vi "Simple Moving Average.vi"(9 "Power v time":cluster{dbl[], dbl[]}(graph), 10 "N point average":i32=5) -> (1 "SMA with Time":cluster{dbl[], dbl[]}(graph), 2 "SMA Graph":dbl[](graph))   [LabVIEW 2017]
uses:
  <vilib>/Analysis/baseanly.llb/Mean (DBL).vi
  <vilib>/Analysis/NI_AALBase.lvlib
panel:
  out "Time":dbl[](array[numeric])
  out "Signal In":dbl[](graph)
  # "Data Input"
  # "Local Data"
  # "Data Output"
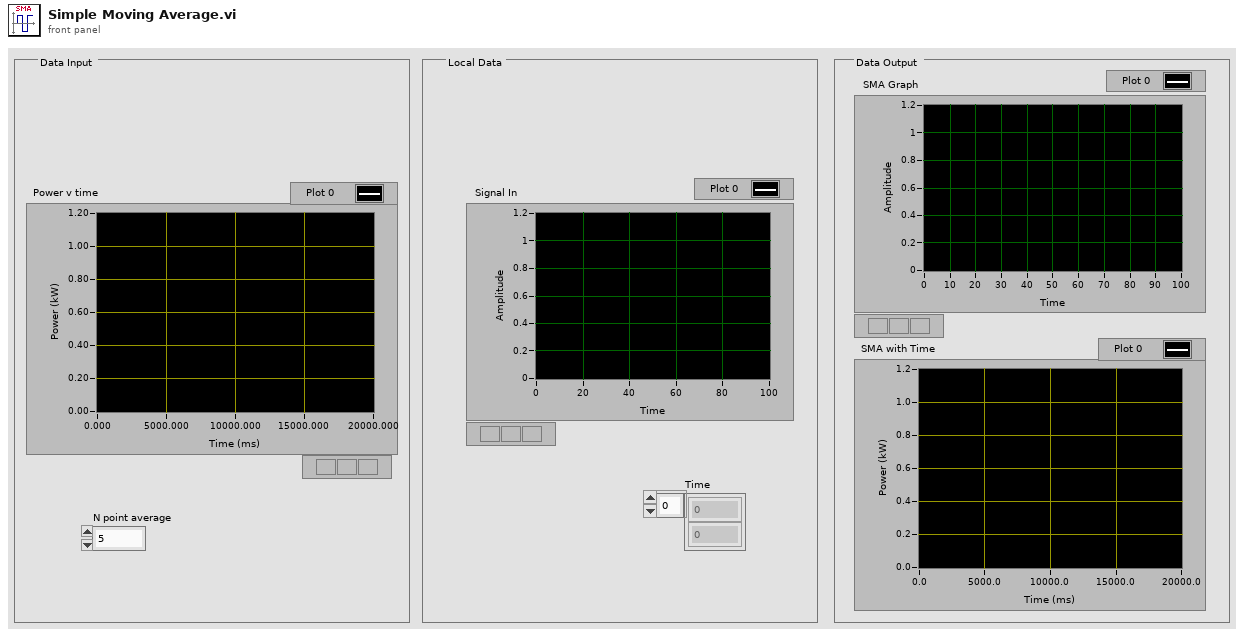
[diagram p1: front panel]
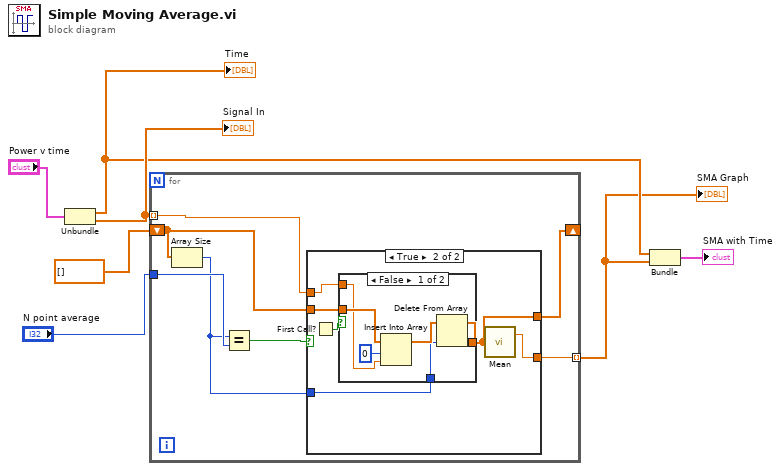
[diagram p0: block diagram]
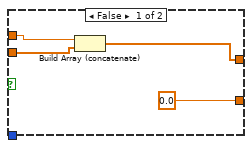
[diagram p2: hidden frame]
diagram:
  n1 = Unbundle("Power v time") -> (w3:dbl[], w6:dbl[])
  "Signal In" <- w6
  "Time" <- w3
  n2 = for {
    tunnel: w6 -> [w11] mode=indexing
    shift-right: [w8] -> _
    shift-left: dbl[] [] -> [w10]
    tunnel: "N point average" -> [w14]
    tunnel: [w12] -> w1 mode=indexing
    n3 = Array Size(array=w10) -> (size(s)=w9:i32)
    n4 = Equal?(x=w9, y=w14) -> (x = y?=w13:bool)
    n5 = case shown="True" w13 {
      tunnel: [0.0 ("Actual Power (kW)") w21] -> w12
      tunnel: w11 -> [w17 w23]
      tunnel: w10 -> [w16 w24]
      tunnel: w9 -> [_ w22]
      tunnel: [w15 w20] -> w8
      frame False {
        n6 = Build Array (concatenate)(w17, w16) -> (w15:dbl[])
      }
      frame True {
        n7 = First Call?() -> (First Call?: T/F=w19:bool)
        n8 = case shown="False" w19 {
          tunnel: w24 -> [w30 w31]
          tunnel: w23 -> [w29 _]
          tunnel: w22 -> [w26 _]
          tunnel: [w25 w31] -> w20
          frame False {
            n9 = Insert Into Array(array=w30, index=0, new element=w29) -> (w27:dbl[])
            n10 = Delete From Array(array=w27, index=w26) -> (array with subset deleted=w25:dbl[])  [unwired: 1 in, 1 out]
          }
          frame True {
          }
        }
        n11 = call-poly <vilib>:"Mean.vi"("X"=w20) -> ("mean"=w21:dbl)  [unwired: 1 out]
      }
    }
  }
  "SMA Graph" <- w1
  n12 = Bundle(w3, w1) -> (→"SMA with Time":cluster{dbl[], dbl[]})  [unwired: 1 in]
